vi "DB_Select.vi"() -> ()   [LabVIEW 2020]
uses:
  <vilib>/addons/database/Connection.llb/DB Tools Open Connec (String).vi
  <vilib>/addons/database/NI_Database_API.lvlib
panel:
  out "Table_ID":string[][](array[string])
  out "data":variant[][](array[variant])
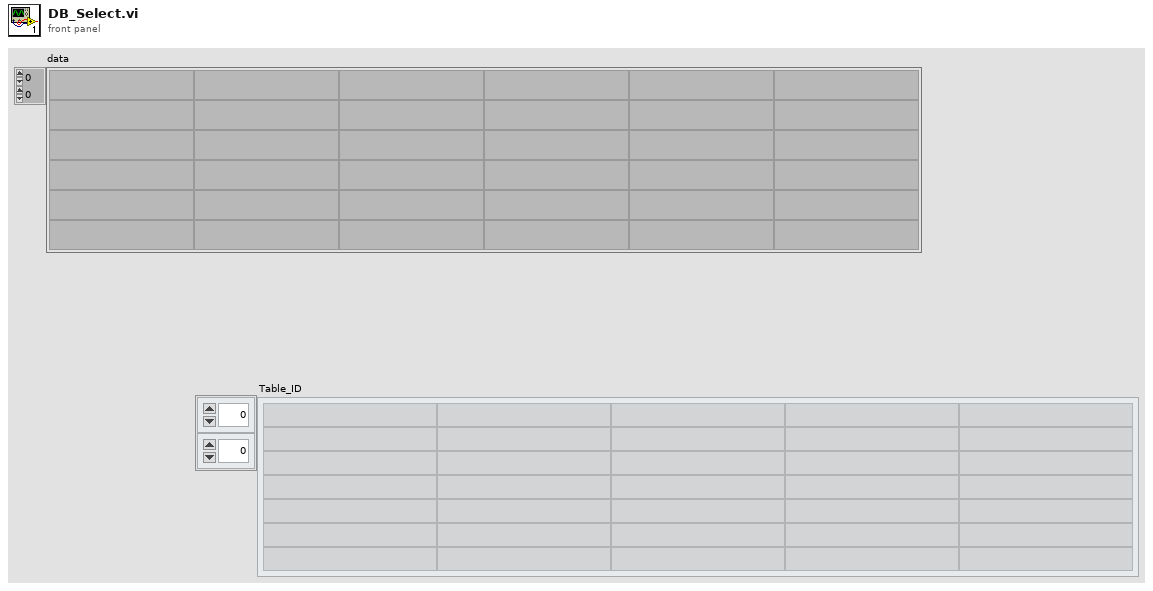
[diagram p1: front panel]
types:
  T1 = typedef "NI_Database_API.lvlib/Conn ObjectReference.ctl" = refnum<k1>
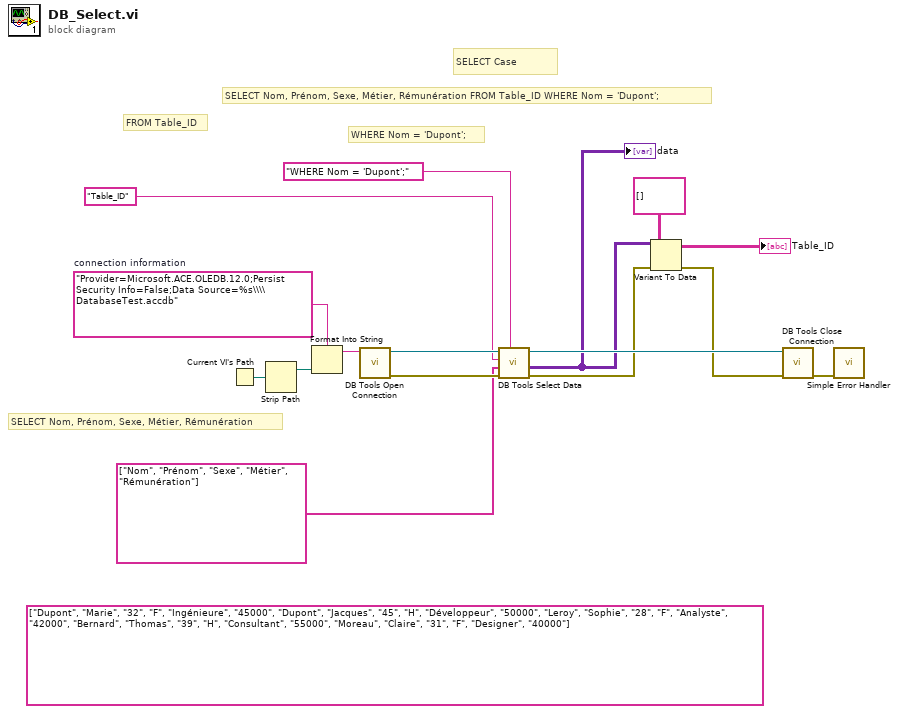
[diagram p0: block diagram]
diagram:
  (unwired) string[][] [["Dupont", "Marie", "32", "F", "Ingénieure", "45000"], ["Dupont", "Jacques", "45", "H", "Développeur", "50000"], ["Leroy", "Sophie", "28", "F", "Analyste", "42000"], ["Bernard", "Thomas", "39", "H", "Consultant", "55000"], ["Moreau", "Claire", "31", "F", "Designer", "40000"]] ("data 2")
  w12 = "Provider=Microsoft.ACE.OLEDB.12.0;Persist Security Info=False;Data Source=%s\\\\DatabaseTest.accdb"  # connection information
  # "WHERE Nom = 'Dupont';"
  # "FROM Table_ID"
  # "SELECT Nom, Prénom, Sexe, Métier, Rémunération"
  # "SELECT Nom, Prénom, Sexe, Métier, Rémunération FROM Table_ID WHERE Nom = 'Dupont';"
  # "SELECT Case"
  n1 = Current VI's Path() -> (path=w16:path)
  n2 = Strip Path(path=w16) -> (stripped path=w13:path)  [unwired: 1 out]
  n3 = Format Into String(format string=w12, w13) -> (resulting string=w14:string)  [unwired: 2 in, 1 out]
  n4 = call-poly <vilib>:"DB Tools Open Connection.vi"("connection information"=w14) -> ("error out"=w11:errorcluster, "connection reference"=w10:T1)  [unwired: 7 in]
  n5 = call <vilib>:"DB Tools Select Data.vi"("condition"="WHERE Nom = 'Dupont';", "error in (no error)"=w11, "columns"=string[] ["Nom", "Prénom", "Sexe", "Métier", "Rémunération"], "table"="Table_ID", "connection reference"=w10) -> ("error out"=w5:errorcluster, "data"=w6:variant[][], "connection reference out"=w8:T1)  [unwired: 1 in]
  "data" <- w6
  n6 = Variant To Data(error in=w5, type=string[][] [], Variant=w6) -> (data=→"Table_ID":string[][], error out=w4:errorcluster)
  n7 = call <vilib>:"DB Tools Close Connection.vi"("error in (no error)"=w4, "connection reference"=w8) -> ("error out"=w15:errorcluster)  [unwired: 5 in]
  n8 = call <vilib>:"Simple Error Handler.vi"("error in (no error)"=w15) -> ()  [unwired: 4 in, 5 out]
